vi "stimulus specification control panel.vi"(8 "error in":errorcluster, 11 "Stimulus Cluster In":T1) -> (0 "error out":errorcluster, 2 "canceled?":bool, 3 "Stimulus Cluster Out":T1)   [LabVIEW 2021]
panel:
  out "Short String":string
  out "Long String":string
  in  "Cancel":bool
  in  "done":bool
  in  "Temporal Parameters":T2
  in  "Spatial Parameters":T3
  in  "Other Parameters":T4
  in  "Stimulant - additional detail":string
  in  "Constant Parameters":T5
  in  "Noise Parameters":T6 {"Full Scale Intensity \n(detector Watts)" format="%#_3p"}
  in  "Stimulant":T7(ring)
  in  "Stimulus Structure":T8(ring)
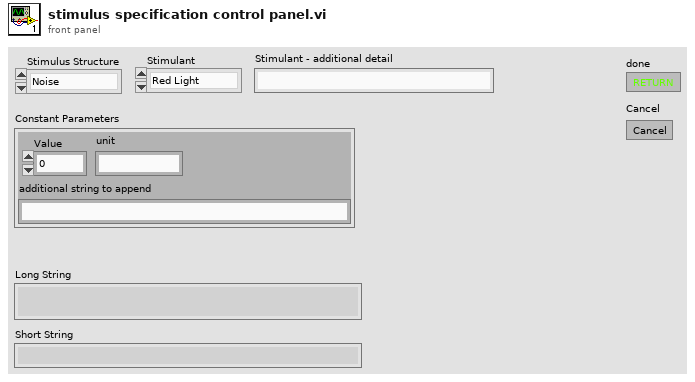
[diagram p1: front panel]
types:
  T1 = cluster{"Stimulus Structure":enum16{"Noise", "Temporal", "Spatial", "Constant", "Other"}, "Stimulant":enum16{"Red Light", "Blue Light", "Green Light", "Odor", "Temperature", "Taste", "Other"}, "Stimulant - additional detail":string, "Noise Parameters":cluster{"Min Val":dbl, "Noise Type":enum16{"Brownian", "Gaussian", "M-Sequence", "Integral of M-Sequence", "Bernoulli", "Uniform", "Other"}, "Max Val":dbl, "Sigma \n(For Gaussian/Brownian)":dbl, "Update Rate (Hz)":dbl, "Full Scale Intensity \n(detector Watts)":dbl, "additional string to append":string, "Other Noise Type":string}, "Temporal Parameters":cluster{"maximum":dbl, "mimimum":dbl, "period (s)":dbl, "Temporal Pattern":enum16{"Triangle", "Sine", "Square", "Other"}, "unit":string, "additional string to append":string, "other pattern":string}, "Spatial Parameters":cluster{"maximum":dbl, "mimimum":dbl, "distance":dbl, "Spatial Pattern":enum16{"XLinear", "YLinear", "Droplet", "Radial", "Other"}, "unit":string, "period_unit":string, "additional string to append":string, "other pattern":string}, "Constant Parameters":cluster{"Value":dbl, "unit":string, "additional string to append":string}, "Other Parameters":cluster{"Long Description of Stimulus And Parameters":string, "Short Description for File Name":string}}
  T2 = cluster{"maximum":dbl, "mimimum":dbl, "period (s)":dbl, "Temporal Pattern":enum16{"Triangle", "Sine", "Square", "Other"}, "unit":string, "additional string to append":string, "other pattern":string}
  T3 = cluster{"maximum":dbl, "mimimum":dbl, "distance":dbl, "Spatial Pattern":enum16{"XLinear", "YLinear", "Droplet", "Radial", "Other"}, "unit":string, "period_unit":string, "additional string to append":string, "other pattern":string}
  T4 = cluster{"Long Description of Stimulus And Parameters":string, "Short Description for File Name":string}
  T5 = cluster{"Value":dbl, "unit":string, "additional string to append":string}
  T6 = cluster{"Min Val":dbl, "Noise Type":enum16{"Brownian", "Gaussian", "M-Sequence", "Integral of M-Sequence", "Bernoulli", "Uniform", "Other"}, "Max Val":dbl, "Sigma \n(For Gaussian/Brownian)":dbl, "Update Rate (Hz)":dbl, "Full Scale Intensity \n(detector Watts)":dbl, "additional string to append":string, "Other Noise Type":string}
  T7 = enum16{"Red Light", "Blue Light", "Green Light", "Odor", "Temperature", "Taste", "Other"}
  T8 = enum16{"Noise", "Temporal", "Spatial", "Constant", "Other"}
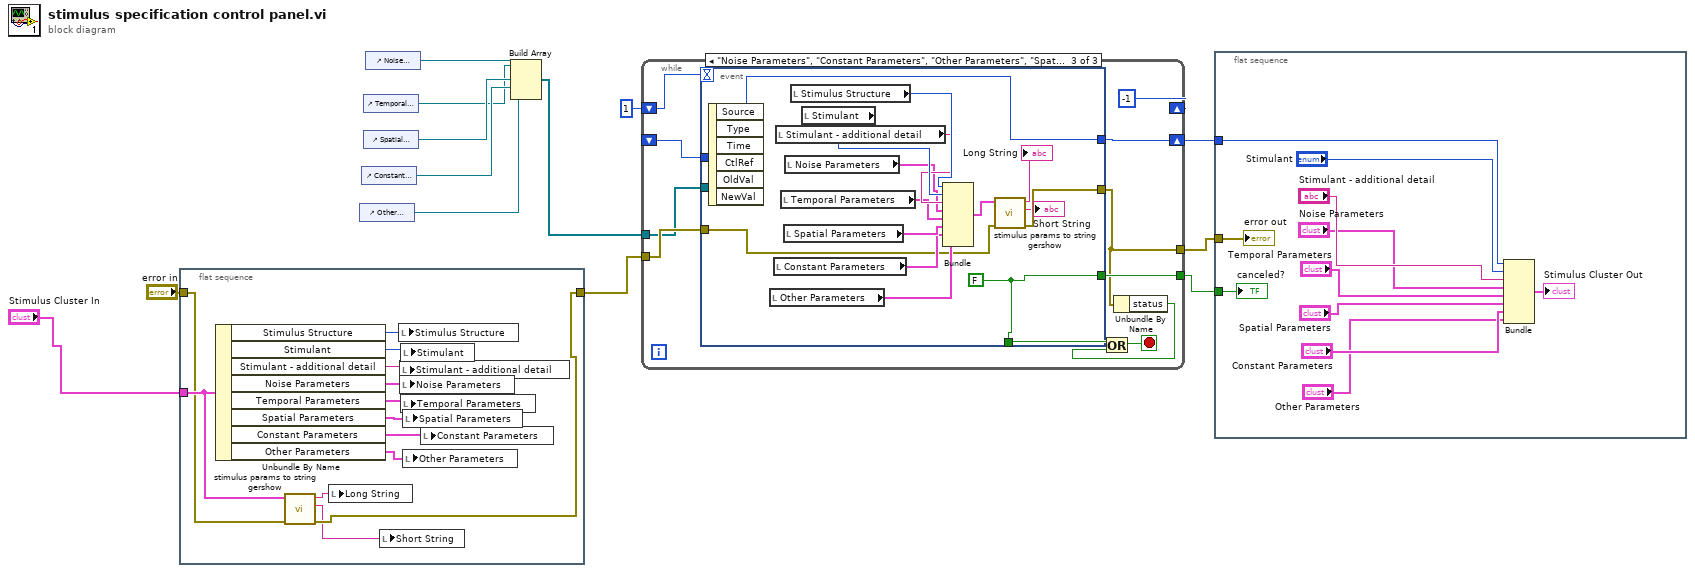
[diagram p0: block diagram]
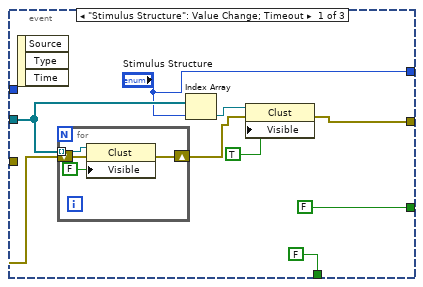
[diagram p2: hidden frame]
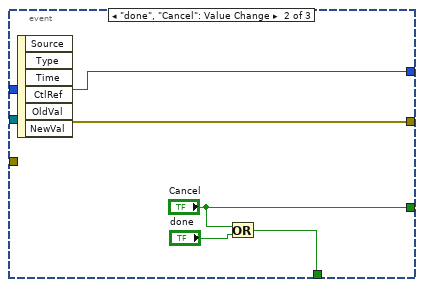
[diagram p3: hidden frame]
diagram:
  n1 = flat-sequence {
    tunnel: "error in" -> [w17]
    tunnel: [w16] -> w3
    tunnel: "Stimulus Cluster In" -> [w18]
    frame #0 {
      n2 = Unbundle By Name(w18) -> ("Stimulus Structure"=w26:T8, "Stimulant"=w25:T7, "Stimulant - additional detail"=w24:string, "Noise Parameters"=w23:T6, "Temporal Parameters"=w22:T2, "Spatial Parameters"=w21:T3, "Constant Parameters"=w20:T5, "Other Parameters"=w19:T4)
      n3 = call "stimulus params to string gershow.vi"("error in"=w17, "Stimulus Cluster In"=w18) -> ("error out"=w16:errorcluster, "Short String"=w14:string, "Long String"=w15:string)  [unwired: 5 in, 2 out]
      n4 = local write "Long String"(w15) -> ()
      n5 = local write "Short String"(w14) -> ()
      n6 = local write "Stimulus Structure"(w26) -> ()
      n7 = local write "Stimulant - additional detail"(w24) -> ()
      n8 = local write "Noise Parameters"(w23) -> ()
      n9 = local write "Stimulant"(w25) -> ()
      n10 = local write "Temporal Parameters"(w22) -> ()
      n11 = local write "Spatial Parameters"(w21) -> ()
      n12 = local write "Other Parameters"(w19) -> ()
      n13 = local write "Constant Parameters"(w20) -> ()
    }
  }
  n14 = control-ref of="Other Parameters"() -> (w10:refnum<vi>)
  n15 = control-ref of="Constant Parameters"() -> (w9:refnum<vi>)
  n16 = control-ref of="Temporal Parameters"() -> (w7:refnum<vi>)
  n17 = control-ref of="Spatial Parameters"() -> (w8:refnum<vi>)
  n18 = control-ref of="Noise Parameters"() -> (w2:refnum<vi>)
  n19 = Build Array(w2, w7, w8, w9, w10) -> (w6:refnum<vi>[])
  n20 = while {
    tunnel: w3 -> [w37]
    tunnel: [w31] -> w13
    shift-right: [-1] -> _
    shift-left: 1 -> [w35]
    tunnel: [w33] -> w11
    tunnel: w6 -> [w32]
    shift-right: [w28] -> w5
    shift-left: _ -> [w27]
    stop <- w30 stop-if-true
    n21 = event shown="[2] \"Noise Parameters\", \"Constant Parameters\", \"Other Parameters\", \"Spatial Parameters\", \"Temporal Parameters\", \"Stimulant - additional detail\", \"Stimulant\": Value Change" {
      selector: _ -> [_ _ _]
      dyn-events: _ -> [_ _ _]
      timeout: w35 -> [_ _ _]
      tunnel: w37 -> [w43 w52 w60]
      tunnel: [w42 w52 w59] -> w31
      tunnel: [FALSE w54 w58] -> w34
      tunnel: [FALSE ("Cancel") "Cancel" w58] -> w33
      tunnel: w32 -> [w39 _ _]
      tunnel: ["Stimulus Structure" w51 w62] -> w28
      tunnel: w27 -> [_ w51 w62]
      event "Stimulus Structure": Value Change; Timeout {
        n22 = event-data() -> ()  [unwired: 1 in, 3 out]
        n23 = for {
          tunnel: w39 -> [w49] mode=indexing
          shift-right: [w48] -> w44
          shift-left: w43 -> [w47]
          n24 = property class="Clust"(reference=w49, error in=w47, "Visible"=FALSE) -> (error out=w48:errorcluster)  [unwired: 1 out]
        }
        n25 = Index Array(array=w39, index="Stimulus Structure") -> (element=w46:refnum<vi>)
        n26 = property class="Clust"(reference=w46, error in=w44, "Visible"=TRUE) -> (error out=w42:errorcluster)  [unwired: 1 out]
      }
      event "done", "Cancel": Value Change {
        n27 = event-data() -> ()  [unwired: 1 in, 6 out]
        n28 = Or(x="Cancel", y="done") -> (x .or. y?=w54:bool)
      }
      event "Noise Parameters", "Constant Parameters", "Other Parameters", "Spatial Parameters", "Temporal Parameters", "Stimulant - additional detail", "Stimulant": Value Change {
        w58 = FALSE ("Cancel")
        n29 = event-data() -> ()  [unwired: 1 in, 6 out]
        n30 = local read "Other Parameters"() -> (w63:T4)
        n31 = local read "Constant Parameters"() -> (w64:T5)
        n32 = local read "Stimulant - additional detail"() -> (w68:string)
        n33 = local read "Temporal Parameters"() -> (w66:T2)
        n34 = local read "Spatial Parameters"() -> (w65:T3)
        n35 = local read "Noise Parameters"() -> (w67:T6)
        n36 = local read "Stimulus Structure"() -> (w70:T8)
        n37 = local read "Stimulant"() -> (w69:T7)
        n38 = Bundle("Stimulus Structure"=w70, "Stimulant"=w69, "Stimulant - additional detail"=w68, "Noise Parameters"=w67, "Temporal Parameters"=w66, "Spatial Parameters"=w65, "Constant Parameters"=w64, "Other Parameters"=w63) -> (w61:T1)  [unwired: 1 in]
        n39 = call "stimulus params to string gershow.vi"("error in"=w60, "Stimulus Cluster In"=w61) -> ("error out"=w59:errorcluster, "Short String"=→"Short String":string, "Long String"=→"Long String":string)  [unwired: 5 in, 2 out]
      }
    }
    n40 = Unbundle By Name(w31) -> ("status"=w29:bool)
    n41 = Or(x=w34, y=w29) -> (x .or. y?=w30:bool)
  }
  n42 = flat-sequence {
    tunnel: w13 -> [w81]
    tunnel: w11 -> [w80]
    tunnel: w5 -> [w72]
    frame #0 {
      n43 = Bundle("Stimulus Structure"=w72, "Stimulant"="Stimulant", "Stimulant - additional detail"="Stimulant - additional detail", "Noise Parameters"="Noise Parameters", "Temporal Parameters"="Temporal Parameters", "Spatial Parameters"="Spatial Parameters", "Constant Parameters"="Constant Parameters", "Other Parameters"="Other Parameters") -> (→"Stimulus Cluster Out":T1)  [unwired: 1 in]
      "error out" <- w81
      "canceled?" <- w80
    }
  }
